vi "error 5100.vi"() -> (0 "error out":errorcluster)   [LabVIEW 2024, in "SN Validator.lvlib"]
uses:
  SN Validator.lvlib
  <vilib>/ErrorRing/Error Ring.xnode
  <vilib>/Utility/error.llb/Error Cluster From Error Code.vi
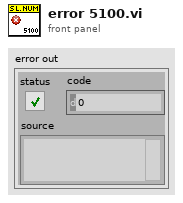
[diagram p1: front panel]
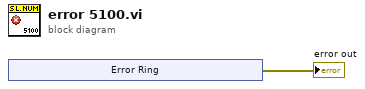
[diagram p0: block diagram]
diagram:
  n1 = xnode "Error Ring"() -> ("error out"=→"error out":errorcluster)
